vi "Test Unicode Tag Vorbis.vi"(8 "error in (no error)":errorcluster) -> (0 "error out":errorcluster, 3 "Pass?":bool)   [LabVIEW 2020]
uses:
  G-Audio/G-Audio.lvlib
  G-Audio/Audio Files/Polymorphic VIs/Get Audio File Tags (Path).vi
  G-Audio/Controls/Text Encoding.ctl
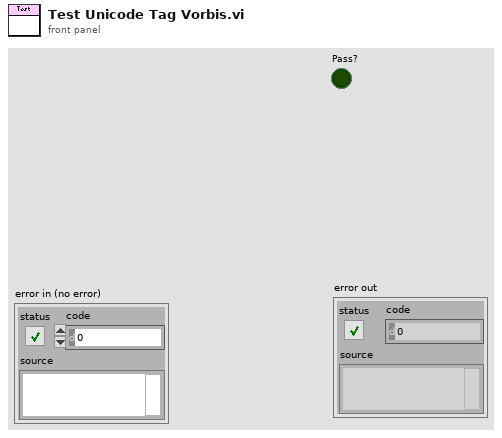
[diagram p1: front panel]
types:
  T1 = typedef "G-Audio.lvlib/Text Encoding.ctl" = enum16{"ASCII", "UTF-8", "UTF-16 LE"}
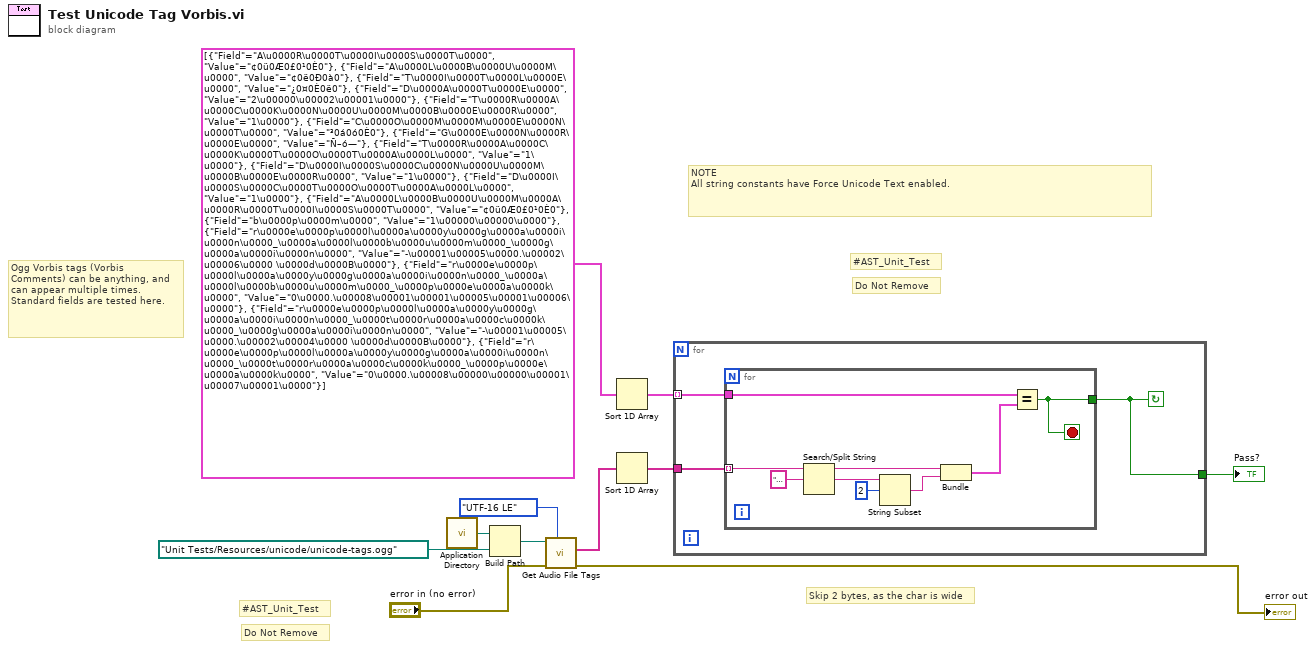
[diagram p0: block diagram]
diagram:
  # "Ogg Vorbis tags (Vorbis Comments) can be anything, and can appear multiple times. Standard fields are tested here."
  # "Skip 2 bytes, as the char is wide"
  # "NOTE\nAll string constants have Force Unicode Text enabled."
  # "Do Not Remove"
  # "#AST_Unit_Test"
  # "Do Not Remove"
  # "#AST_Unit_Test"
  n1 = call <vilib>:"Application Directory.vi"() -> ("Application Directory"=w11:path)
  n2 = Build Path(base path=w11, name or relative path=path "Unit Tests/Resources/unicode/unicode-tags.ogg" ("Path")) -> (appended path=w9:path)
  n3 = call-poly "Get Audio File Tags.vi"("Encoding (ASCII)"=Text_Encoding."UTF-16 LE", "error in (no error)"="error in (no error)", "Path In"=w9) -> ("error out"=→"error out":errorcluster, "Tags"=w8:string[])  [unwired: 6 in, 1 out]
  n4 = Sort 1D Array(array=cluster{"Field":string, "Value":string}[] [{"Field"="A\u0000R\u0000T\u0000I\u0000S\u0000T\u0000", "Value"="¢0ü0Æ0£0¹0È0"}, {"Field"="A\u0000L\u0000B\u0000U\u0000M\u0000", "Value"="¢0ë0Ð0à0"}, {"Field"="T\u0000I\u0000T\u0000L\u0000E\u0000", "Value"="¿0¤0È0ë0"}, {"Field"="D\u0000A\u0000T\u0000E\u0000", "Value"="2\u00000\u00002\u00001\u0000"}, {"Field"="T\u0000R\u0000A\u0000C\u0000K\u0000N\u0000U\u0000M\u0000B\u0000E\u0000R\u0000", "Value"="1\u0000"}, {"Field"="C\u0000O\u0000M\u0000M\u0000E\u0000N\u0000T\u0000", "Value"="³0á0ó0È0"}, {"Field"="G\u0000E\u0000N\u0000R\u0000E\u0000", "Value"="Ñ–ó—"}, {"Field"="T\u0000R\u0000A\u0000C\u0000K\u0000T\u0000O\u0000T\u0000A\u0000L\u0000", "Value"="1\u0000"}, {"Field"="D\u0000I\u0000S\u0000C\u0000N\u0000U\u0000M\u0000B\u0000E\u0000R\u0000", "Value"="1\u0000"}, {"Field"="D\u0000I\u0000S\u0000C\u0000T\u0000O\u0000T\u0000A\u0000L\u0000", "Value"="1\u0000"}, {"Field"="A\u0000L\u0000B\u0000U\u0000M\u0000A\u0000R\u0000T\u0000I\u0000S\u0000T\u0000", "Value"="¢0ü0Æ0£0¹0È0"}, {"Field"="b\u0000p\u0000m\u0000", "Value"="1\u00000\u00000\u0000"}, {"Field"="r\u0000e\u0000p\u0000l\u0000a\u0000y\u0000g\u0000a\u0000i\u0000n\u0000_\u0000a\u0000l\u0000b\u0000u\u0000m\u0000_\u0000g\u0000a\u0000i\u0000n\u0000", "Value"="-\u00001\u00005\u0000.\u00002\u00006\u0000 \u0000d\u0000B\u0000"}, {"Field"="r\u0000e\u0000p\u0000l\u0000a\u0000y\u0000g\u0000a\u0000i\u0000n\u0000_\u0000a\u0000l\u0000b\u0000u\u0000m\u0000_\u0000p\u0000e\u0000a\u0000k\u0000", "Value"="0\u0000.\u00008\u00001\u00001\u00005\u00001\u00006\u0000"}, {"Field"="r\u0000e\u0000p\u0000l\u0000a\u0000y\u0000g\u0000a\u0000i\u0000n\u0000_\u0000t\u0000r\u0000a\u0000c\u0000k\u0000_\u0000g\u0000a\u0000i\u0000n\u0000", "Value"="-\u00001\u00005\u0000.\u00002\u00004\u0000 \u0000d\u0000B\u0000"}, {"Field"="r\u0000e\u0000p\u0000l\u0000a\u0000y\u0000g\u0000a\u0000i\u0000n\u0000_\u0000t\u0000r\u0000a\u0000c\u0000k\u0000_\u0000p\u0000e\u0000a\u0000k\u0000", "Value"="0\u0000.\u00008\u00000\u00000\u00001\u00007\u00001\u0000"}]) -> (sorted array=w7:cluster{"Field":string, "Value":string}[])
  n5 = Sort 1D Array(array=w8) -> (sorted array=w2:string[])
  n6 = for {
    tunnel: w2 -> [w14]
    tunnel: w7 -> [w12] mode=indexing
    tunnel: [w13] -> w4
    stop <- w13 continue-if-true
    n7 = for {
      tunnel: w14 -> [w15] mode=indexing
      tunnel: [w17] -> w13
      tunnel: w12 -> [w18]
      stop <- w17 stop-if-true
      n8 = Search/Split String(string=w15, search string/char (-)="=\u0000") -> (substring before match=w16:string, match + rest of string=w21:string)  [unwired: 1 in, 1 out]
      n9 = String Subset(string=w21, offset (0)=2) -> (substring=w19:string)  [unwired: 1 in]
      n10 = Bundle("string"=w16, "string"=w19) -> (w22:cluster{"string":string, "string":string})  [unwired: 1 in]
      n11 = Equal?(x=w18, y=w22) -> (x = y?=w17:bool)
    }
  }
  "Pass?" <- w4
